vi "ListFiles.vi"() -> ()   [LabVIEW 8.6]
uses:
  EDSDK-Labview.llb/kEdsImageSrcs.ctl
  EDSDK-Labview.llb/kEdsTargetImageTypes.ctl
  EDSDK-Labview.llb/kEdsProperties.ctl
  EDSDK-Labview.llb/EdsImageQuality.ctl
  EDSDK-Labview.llb/kEdsStorageType.ctl
  EDSDK-Labview.llb/EdsAccess.ctl
  EDSDK-Labview.llb/kEdsImageTypes.ctl
panel:
  out "timing details":cluster{"FileName":string, u32, "Numeric":dbl}[](array[cluster])
  in  "Image Type":T1 items=["Grayscale (U8)", "Grayscale (I16)", "Grayscale (SGL)", "Complex (CSG)", "RGB (U32)", "HSL (U32)", "RGB (U64)", "Grayscale (U16)"]
  out "dt":u32
  out "current file":string
  in  "full/thumbnail":bool
  in  "stop":bool
  out "Image Out":T2(plugin-control)
  out "files":T4(array[cluster]) {"format" items=["Unknown", "Jpeg", "CRW", "RAW", "CR2", "MOVwithTHM", "MOVwithoutTHM"]}
  out "subfolders":T6(array[cluster]) {"format" items=["Unknown", "Jpeg", "TIFF", "TIFF16", "RGB", "RGB16", "DIB"]}
  out "folders":T6(array[cluster]) {"format" items=["Unknown", "Jpeg", "TIFF", "TIFF16", "RGB", "RGB16", "DIB"]}
  out "disks":T9(array[cluster]) {"kEdsStorageType" items=["Non", "CF", "SD", "HD"]; "EdsAccess" items=["ReadOnly", "WriteOnly", "ReadWrite", "Error"]}
  out "cameras":u32
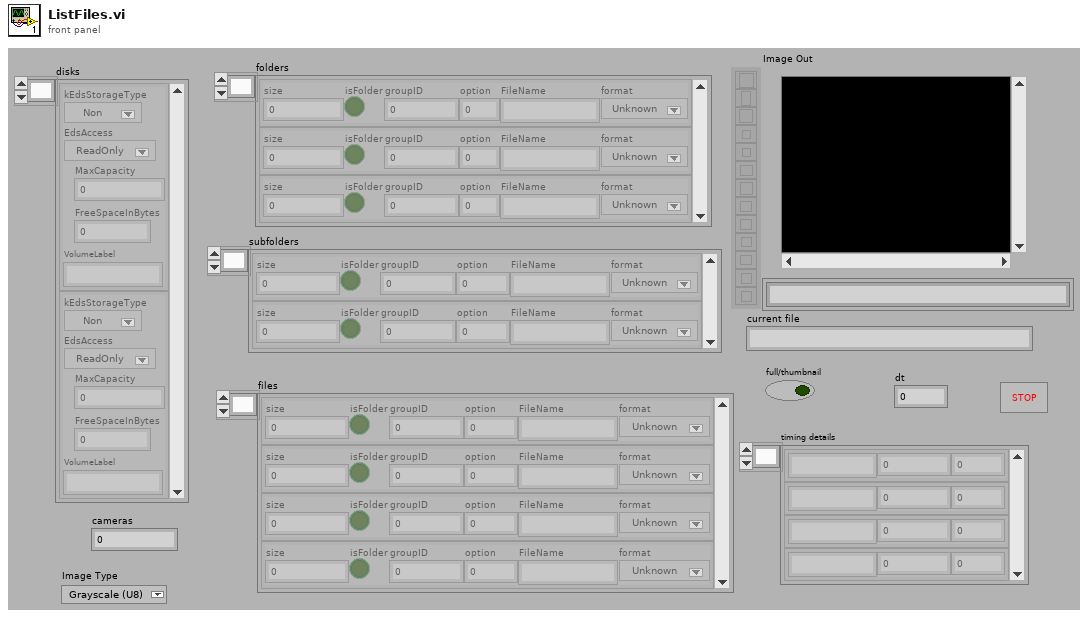
[diagram p1: front panel]
types:
  T1 = typedef "Image Type" = u32
  T2 = typedef "IMAQ Image.ctl" = refnum<image>
  T3 = typedef "kEdsImageTypes.ctl" = u32
  T4 = cluster{"size":u32, "isFolder":bool, "groupID":u32, "option":u32, "FileName":string, "format":T3}[]
  T5 = typedef "kEdsTargetImageTypes.ctl" = u32
  T6 = cluster{"size":u32, "isFolder":bool, "groupID":u32, "option":u32, "FileName":string, "format":T5}[]
  T7 = typedef "kEdsStorageType.ctl" = u32
  T8 = typedef "EdsAccess.ctl" = u32
  T9 = cluster{"kEdsStorageType":T7, "EdsAccess":T8, "MaxCapacity":u64, "FreeSpaceInBytes":u64, "VolumeLabel":string}[]
  T10 = cluster{"kEdsStorageType":T7, "EdsAccess":T8, "MaxCapacity":u64, "FreeSpaceInBytes":u64, "VolumeLabel":string}
  T11 = typedef "EdsImageQuality.ctl" = u32
  T12 = typedef "kEdsProperties.ctl" = u32
  T13 = typedef "kEdsImageSrcs.ctl" = u32
  T14 = typedef "EdsImageInfo.ctl" = cluster{"width":u32, "height":u32, "# components":u32, "bit depth":u32, "rect":u32[], "reserved 1":u32, "reserved 2":u32}
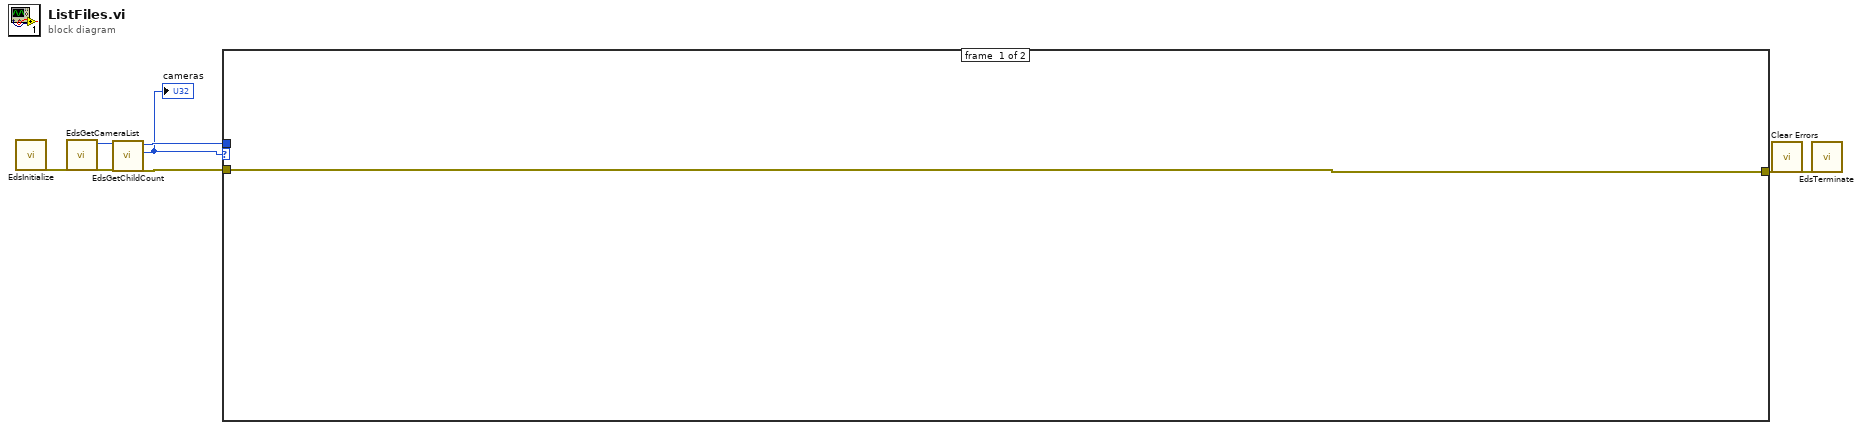
[diagram p0: block diagram]
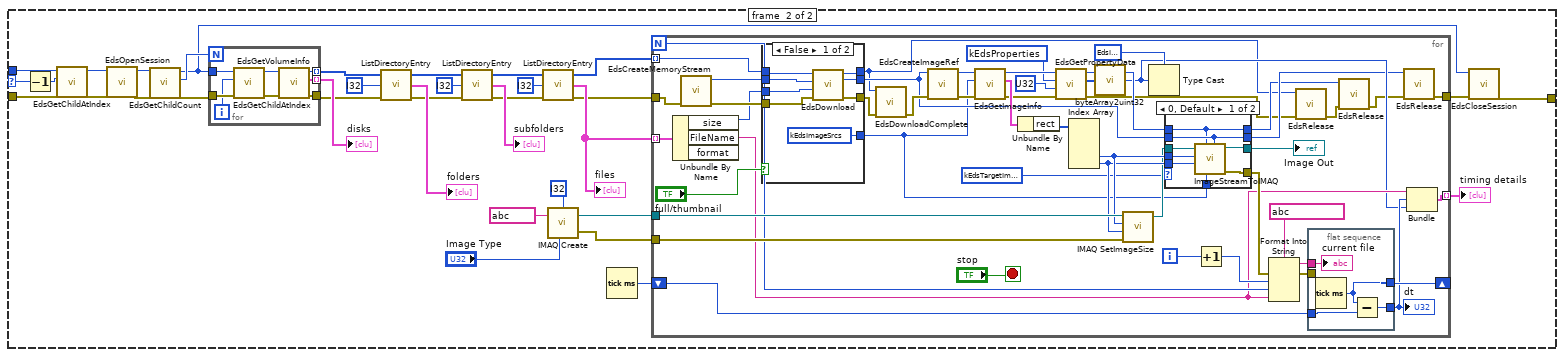
[diagram p2: hidden frame]
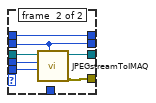
[diagram p3: hidden frame]
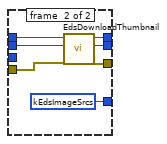
[diagram p4: hidden frame]
diagram:
  n1 = call "EdsInitialize.vi"() -> ("error out"=w8:errorcluster)  [unwired: 11 in]
  n2 = call "EdsGetCameraList.vi"("error in"=w8) -> ("error out"=w4:errorcluster, "outCameraListRef"=w5:u32)  [unwired: 9 in]
  n3 = call "EdsGetChildCount.vi"("error in"=w4, "inRef"=w5) -> ("error out"=w3:errorcluster, "count"=w1:u32, "inRef dup"=w2:u32)  [unwired: 7 in]
  "cameras" <- w1
  n4 = case shown="1, Default" w1 {
    selector: w1 -> [_ w39]
    tunnel: w2 -> [_ w41]
    tunnel: w3 -> [w9 w40]
    tunnel: [w9 w38] -> w6
    frame #0 {
    }
    frame #1 {
      n5 = Decrement(x=w39) -> (x-1=w44:u32)
      n6 = call "EdsGetChildAtIndex.vi"("error in"=w40, "index"=w44, "inRef"=w41) -> ("error out"=w42:errorcluster, "outRef"=w43:u32)  [unwired: 7 in]
      n7 = call "EdsOpenSession.vi"("error in"=w42, "inCameraRef"=w43) -> ("error out"=w36:errorcluster, "inCameraRef dup"=w37:u32)  [unwired: 8 in]
      n8 = call "EdsGetChildCount.vi"("error in"=w36, "inRef"=w37) -> ("error out"=w35:errorcluster, "count"=w34:u32, "inRef dup"=w33:u32)  [unwired: 7 in]
      n9 = for {
        N: w34 -> [_]
        tunnel: w33 -> [w136]
        tunnel: w35 -> [w135]
        tunnel: [w131] -> w30
        tunnel: [w130] -> w32 mode=indexing
        tunnel: [w129] -> w31 mode=indexing
        i -> [w134]
        n10 = call "EdsGetChildAtIndex.vi"("error in"=w135, "index"=w134, "inRef"=w136) -> ("error out"=w132:errorcluster, "outRef"=w133:u32)  [unwired: 7 in]
        n11 = call "EdsGetVolumeInfo.vi"("error in"=w132, "inVolumeRef"=w133) -> ("error out"=w131:errorcluster, "VolumeInfo"=w130:T10, "inVolumeRef dup"=w129:u32)  [unwired: 7 in]
      }
      "disks" <- w32
      n12 = call "ListDirectoryEntry.vi"("error out 2"=w30, "entry to descend"=i32 ? ("index"), "Dir items at this level"=w31) -> ("error out"=w27:errorcluster, "dir List"=→"folders":T6, "inner items refs"=w26:u32[])
      n13 = call "ListDirectoryEntry.vi"("error out 2"=w27, "entry to descend"=i32 ?, "Dir items at this level"=w26) -> ("error out"=w21:errorcluster, "dir List"=→"subfolders":T6, "inner items refs"=w22:u32[])
      n14 = call "ListDirectoryEntry.vi"("error out 2"=w21, "entry to descend"=i32 ?, "Dir items at this level"=w22) -> ("error out"=w18:errorcluster, "dir List"=w19:T6, "inner items refs"=w20:u32[])
      "files" <- w19
      n15 = call "IMAQ Create"("Border Size"=i32 ?, "Image Name"=string ?, "Image Type"="Image Type") -> ("New Image"=w13:T2, "error out"=w12:errorcluster)  [unwired: 2 in]
      n16 = Tick Count (ms)() -> (millisecond timer value=w11:u32)
      n17 = for {
        N -> [w73]
        tunnel: w20 -> [w80] mode=indexing
        tunnel: w19 -> [w81] mode=indexing
        tunnel: w18 -> [w94]
        tunnel: [w53] -> w17
        tunnel: w13 -> [w87]
        tunnel: w12 -> [w86]
        shift-right: [w69] -> _
        shift-left: w11 -> [w68]
        tunnel: [w64] -> w10 mode=indexing
        i -> [w75]
        stop <- "stop" stop-if-true
        w56 = T11 ? items=["LJ", "M1J", "M2J", "SJ", "LJF", "LJN", "MJF", "MJN", "SJF", "SJN", "S1JF", "S1JN", "S2JF", "S3JF", "LR", "LRLJF", "LRLJN", "LRMJF", "LRMJN", "LRSJF", "LRSJN", "LRS1JF", "LRS1JN", "LRS2JF", "LRS3JF", "LRLJ", "LRM1J", "LRM2J", "LRSJ", "MR", "MRLJF", "MRLJN", "MRMJF", "MRMJN", "MRSJF", "MRSJN", "MRS1JF", "MRS1JN", "MRS2JF", "MRS3JF", "MRLJ", "MRM1J", "MRM2J", "MRSJ", "SR", "SRLJF", "SRLJN", "SRMJF", "SRMJN", "SRSJF", "SRSJN", "SRS1JF", "SRS1JN", "SRS2JF", "SRS3JF", "SRLJ", "SRM1J", "SRM2J", "SRSJ", "Unknown"] ("EdsImageQuality")
        w57 = T12 ? items=["Unknown", "ProductName", "BodyID", "OwnerName", "MakerName", "DateTime", "FirmwareVersion", "BatteryLevel", "CFn", "SaveTo", "CurrentStorage", "CurrentFolder", "MyMenu", "BatteryQuality", "HDDirectoryStructure", "ImageQuality", "JpegQuality", "Orientation", "ICCProfile", "FocusInfo", "DigitalExposure", "WhiteBalance", "ColorTemperature", "WhiteBalanceShift", "Contrast", "ColorSaturation", "ColorTone", "Sharpness", "ColorSpace", "ToneCurve", "PhotoEffect", "FilterEffect", "ToningEffect", "ParameterSet", "ColorMatrix", "PictureStyle", "PictureStyleDesc", "ETTL2Mode", "PictureStyleCaption", "Linear", "ClickWBPoint", "WBCoeffs", "GPSVersionID", "GPSLatitudeRef", "GPSLatitude", "GPSLongitudeRef", "GPSLongitude", "GPSAltitudeRef", "GPSAltitude", "GPSTimeStamp", "GPSSatellites", "GPSStatus", "GPSMapDatum", "GPSDateStamp", "AtCapture_Flag", "AEMode", "DriveMode", "ISOSpeed", "MeteringMode", "AFMode", "Av", "Tv", "ExposureCompensation", "FlashCompensation", "FocalLength", "AvailableShots", "Bracket", "WhiteBalanceBracket", "LensName", "AEBracket", "FEBracket", "ISOBracket", "NoiseReduction", "FlashOn", "RedEye", "FlashMode", "LensStatus", "Artist", "Copyright", "DepthOfField", "EFCompensation", "Evf_OutputDevice", "Evf_Mode", "Evf_WhiteBalance", "Evf_ColorTemperature", "Evf_DepthOfFieldPreview", "Evf_Zoom", "Evf_ZoomPosition", "Evf_FocusAid", "Evf_Histogram", "Evf_ImagePosition", "Evf_HistogramStatus", "Evf_AFMode", "Evf_CoordinateSystem", "Evf_ZoomRect"] ("inPropertyID")
        w63 = T5 ? items=["Unknown", "Jpeg", "TIFF", "TIFF16", "RGB", "RGB16", "DIB"] ("format")
        n18 = Unbundle By Name(w81) -> ("size"=w82:u32, "FileName"=w66:string)  [unwired: 1 out]
        n19 = call "EdsCreateMemoryStream.vi"("error in"=w94) -> ("error out"=w93:errorcluster, "outStreamRef"=w92:u32)  [unwired: 9 in]
        n20 = case shown="False" "full/thumbnail" {
          tunnel: w80 -> [w119 w128]
          tunnel: w93 -> [w121 w127]
          tunnel: w92 -> [w116 w126]
          tunnel: [w120 w125] -> w91
          tunnel: [w118 w124] -> w46
          tunnel: [w117 w123] -> w52
          tunnel: w82 -> [w115 _]
          tunnel: [w114 w122] -> w45
          frame #0 {
            w114 = T13 ? items=["FullView", "Thumbnail", "Preview", "RAWThumbnail", "RAWFullView"] ("inImageSource")
            n21 = call "EdsDownload.vi"("error in"=w121, "inReadSize"=w115, "outStreamRef"=w116, "inDirItemRef"=w119) -> ("error out"=w120:errorcluster, "outStreamRef dup"=w117:u32, "inDirItemRef dup"=w118:u32)  [unwired: 5 in]
          }
          frame #1 {
            w122 = T13 ? items=["FullView", "Thumbnail", "Preview", "RAWThumbnail", "RAWFullView"] ("inImageSource")
            n22 = call "EdsDownloadThumbnail.vi"("error in"=w127, "outStreamRef"=w126, "inDirItemRef"=w128) -> ("error out"=w125:errorcluster, "outStreamRef dup"=w123:u32, "inDirItemRef dup"=w124:u32)  [unwired: 6 in]
          }
        }
        n23 = call "EdsDownloadComplete.vi"("error in"=w91, "inDirItemRef"=w46) -> ("error out"=w90:errorcluster)  [unwired: 9 in]
        n24 = call "EdsCreateImageRef.vi"("error in"=w90, "inStreamRef"=w52) -> ("error out"=w88:errorcluster, "outImageRef"=w89:u32)  [unwired: 8 in]
        n25 = call "EdsGetImageInfo.vi"("error in"=w88, "inImageSource"=w45, "inImageRef"=w89) -> ("error out"=w60:errorcluster, "outImageInfo"=w84:T14, "inImageRef dup"=w61:u32)  [unwired: 6 in]
        n26 = Unbundle By Name(w84) -> ("rect"=w79:u32[])
        n27 = call "EdsGetPropertyData.vi"("error in"=w60, "inPropertySize"=u32 ?, "inPropertyID"=w57, "inRef"=w61) -> ("error out"=w47:errorcluster, "outPropertyData"=w55:u8[], "inRef dup"=w59:u32)  [unwired: 5 in]
        n28 = Index Array(array=w79) -> (element #3=w78:u32, element #4=w77:u32)  [unwired: 4 in, 2 out]
        n29 = call "byteArray2uint32.vi"("byteArray"=w55) -> ("uint32"=w54:u32)
        n30 = call "IMAQ SetImageSize"("error in (no error)"=w86, "Y Resolution"=w77, "X Resolution"=w78, "Image"=w87) -> ("Image Out"=w67:T2)  [unwired: 1 in, 1 out]
        n31 = Type Cast(type=w56, x=w54) -> ()  [unwired: 1 out]
        n32 = case shown="0, Default" w63 {
          tunnel: w67 -> [w100 w109]
          tunnel: [w102 w108] -> w85
          tunnel: w52 -> [w97 w104]
          tunnel: w78 -> [w99 w107]
          tunnel: w77 -> [w98 w106]
          tunnel: [w101 w105] -> w70
          tunnel: w59 -> [w96 w103]
          tunnel: [w97 w104] -> w51
          tunnel: [w96 w103] -> w49
          tunnel: w45 -> [w95 _]
          frame #0 {
            n33 = call "ImageStreamToIMAQ.vi"("inStreamRef"=w97, "inImageRef"=w96, "inImageSource (Thumbnail for evf)"=w95, "height"=w98, "width"=w99, "Image"=w100) -> ("error out"=w101:errorcluster, "Image Out"=w102:T2)  [unwired: 4 in]
          }
          frame #1 {
            n34 = call "JPEGstreamToIMAQ.vi"("inStream"=w104, "height"=w106, "width"=w107, "Image"=w109) -> ("error out"=w105:errorcluster, "Image Out"=w108:T2)  [unwired: 3 in]
          }
        }
        "Image Out" <- w85
        n35 = Increment(x=w75) -> (x+1=w74:i32)
        n36 = Format Into String(format string=string ?, error in=w70, w74, w73, w66) -> (resulting string=w71:string, error out=w62:errorcluster)  [unwired: 1 in]
        n37 = call "EdsRelease.vi"("error in"=w47, "inRef"=w46) -> ("error out"=w48:errorcluster)  [unwired: 7 in, 2 out]
        n38 = flat-sequence {
          tunnel: w71 -> [w113]
          tunnel: [w112] -> w69
          tunnel: w68 -> [w111]
          tunnel: [w110] -> w65
          tunnel: w62 -> [_]
          frame #0 {
            n39 = Tick Count (ms)() -> (millisecond timer value=w112:u32)
            n40 = Subtract(x=w112, y=w111) -> (x-y=w110:u32)
            "current file" <- w113
          }
        }
        n41 = call "EdsRelease.vi"("error in"=w48, "inRef"=w49) -> ("error out"=w50:errorcluster)  [unwired: 7 in, 2 out]
        n42 = call "EdsRelease.vi"("error in"=w50, "inRef"=w51) -> ("error out"=w53:errorcluster)  [unwired: 7 in, 2 out]
        n43 = Bundle("FileName"=w66, w65, "uint32"=w54) -> (w64:cluster{"FileName":string, u32, "uint32":u32})  [unwired: 1 in]
        "dt" <- w65
      }
      "timing details" <- w10
      n44 = call "EdsCloseSession.vi"("error in"=w17, "inCameraRef"=w33) -> ("error out"=w38:errorcluster)  [unwired: 8 in, 1 out]
    }
  }
  n45 = call <vilib>:"Clear Errors.vi"("error in (no error)"=w6) -> ("error out"=w7:errorcluster)  [unwired: 6 in]
  n46 = call "EdsTerminate.vi"("error in"=w7) -> ()  [unwired: 10 in, 1 out]
